vi "BLM_SetToValue.vi"(4 "error in (no error)":errorcluster, 5 "Position":dbl min=-2147483647.0 max=2147483647.0 format="%#_10g", 6 "Motor Address":string="0", 7 "Port Address":refnum<visa-resource-name>) -> (0 "error out":errorcluster, 3 "Port Address Out":refnum<visa-resource-name>)   [LabVIEW 2020]
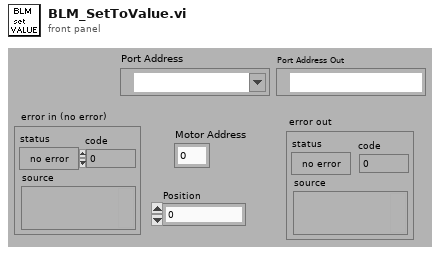
[diagram p1: front panel]
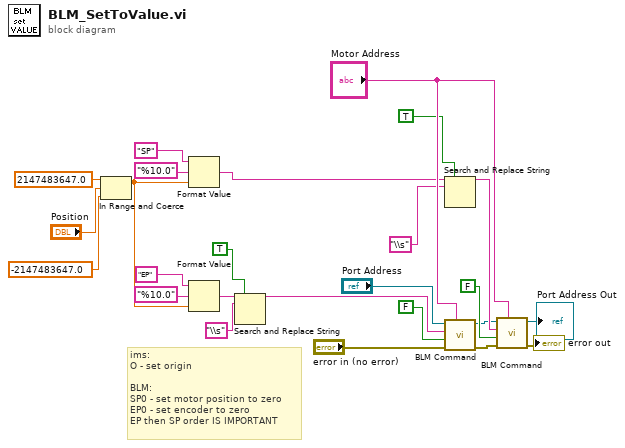
[diagram p0: block diagram]
diagram:
  # "ims:\nO - set origin\n\nBLM:\nSP0 - set motor position to zero\nEP0 - set encoder to zero\nEP then SP order IS IMPORTANT"
  n1 = In Range and Coerce(upper limit=2147483647.0 ("x"), x="Position", lower limit=-2147483647.0) -> (coerced(x)=w18:dbl)  [unwired: 1 out]
  n2 = Format Value(string ("")="SP", format string="%10.0", value (0)=w18) -> (output string=w11:string)
  n3 = Format Value(string ("")="EP", format string="%10.0", value (0)=w18) -> (output string=w8:string)
  n4 = Search and Replace String(replace all?=TRUE ("replace all? (F)"), input string=w8, search string="\\s") -> (result string=w7:string)  [unwired: 5 in, 3 out]
  n5 = Search and Replace String(replace all?=TRUE ("replace all? (F)"), input string=w11, search string="\\s") -> (result string=w12:string)  [unwired: 5 in, 3 out]
  n6 = call "BLM Command.vi"("Motor Address"="Motor Address", "error in (no error)"="error in (no error)", "Read Echo?"=FALSE, "Command"=w7, "Port Address"="Port Address") -> ("error out"=w16:errorcluster, "Port Address Out"=w2:refnum<visa-resource-name>)  [unwired: 1 in, 3 out]
  n7 = call "BLM Command.vi"("Motor Address"="Motor Address", "error in (no error)"=w16, "Read Echo?"=FALSE, "Command"=w12, "Port Address"=w2) -> ("error out"=→"error out":errorcluster, "Port Address Out"=→"Port Address Out":refnum<visa-resource-name>)  [unwired: 1 in, 3 out]
